vi "testStopServer.vi"(8 "error in (no error)":errorcluster) -> (0 "error out":errorcluster)   [LabVIEW 2018]
doc: "Test the stopServer.vi."
uses:
  src/FactoryTcpServer/FactoryTcpServer.lvclass
  src/TcpServer/TcpServer.lvclass/TcpServer.ctl
  src/TcpServerTel/TcpServerTel.lvclass/TcpServerTel.ctl
  src/TcpServerCmd/TcpServerCmd.lvclass
  home/pcortes/Documents/github/ts_labview_tcp_json/src/TcpServerBase/TcpServerBase.lvclass
  src/TcpServerTel/TcpServerTel.lvclass
  <vilib>/addons/_JKI Toolkits/Caraya/classes/Assert/Assert False.vi
  <vilib>/addons/_JKI Toolkits/Caraya/classes/Assert/Assert True.vi
  <vilib>/addons/_JKI Toolkits/Caraya/classes/Test/Test.lvclass
  <vilib>/addons/_JKI Toolkits/Caraya/classes/Assert/Assert.lvclass
  src/TcpServer/TcpServer.lvclass
  src/TcpServerBase/TcpServerBase.lvclass
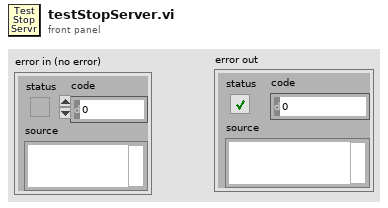
[diagram p1: front panel]
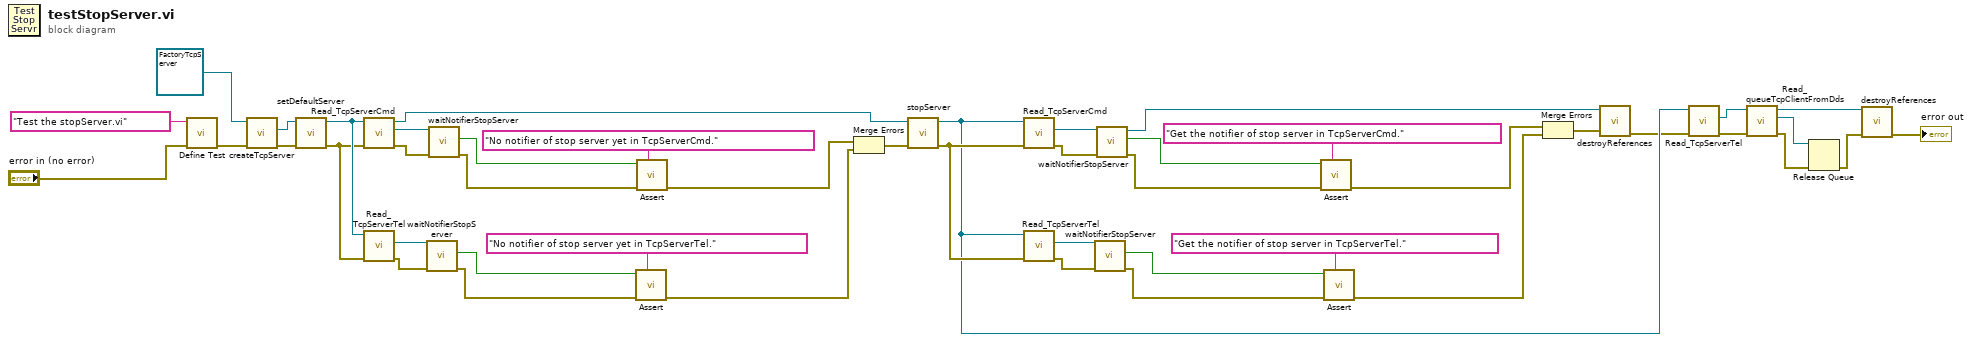
[diagram p0: block diagram]
diagram:
  n1 = call <vilib>:"Define Test.vi"("error in (no error)"="error in (no error)", "Label (VI Title)"="Test the stopServer.vi") -> ("error out"=w15:errorcluster)  [unwired: 9 in]
  n2 = call "createTcpServer.vi"("error in (no error)"=w15, "FactoryTcpServer in"=refnum<class "FactoryTcpServer.lvclass"> refnum) -> ("error out"=w14:errorcluster, "TcpServer out"=w13:refnum<class "TcpServer.lvclass">)  [unwired: 7 in, 1 out]
  n3 = call "setDefaultServer.vi"("error in (no error)"=w14, "TcpServer.lvclass"=w13) -> ("error out"=w42:errorcluster, "tcpServer out"=w43:refnum<class "TcpServer.lvclass">)  [unwired: 8 in]
  n4 = call "Read_TcpServerCmd.vi"("error in (no error)"=w42, "TcpServer in"=w43) -> ("error out"=w39:errorcluster, "TcpServerCmd.lvclass"=w40:refnum<class "TcpServerCmd.lvclass">, "TcpServer out"=w44:refnum<class "TcpServer.lvclass">)  [unwired: 7 in]
  n5 = call "Read_TcpServerTel.vi"("error in (no error)"=w42, "TcpServer in"=w43) -> ("error out"=w37:errorcluster, "TcpServerTel.lvclass"=w38:refnum<class "TcpServerTel.lvclass">)  [unwired: 7 in, 1 out]
  n6 = call "waitNotifierStopServer.vi"("error in (no error)"=w37, "TcpServerBase in"=w38) -> ("error out"=w32:errorcluster, "stopServer"=w33:bool)  [unwired: 7 in, 1 out]
  n7 = call "waitNotifierStopServer.vi"("error in (no error)"=w39, "TcpServerBase in"=w40) -> ("error out"=w31:errorcluster, "stopServer"=w36:bool)  [unwired: 7 in, 1 out]
  n8 = call-poly <vilib>:"Assert.vi"("Label"="No notifier of stop server yet in TcpServerTel.", "error in (no error)"=w32, "False?"=w33) -> ("error out"=w29:errorcluster)  [unwired: 8 in]
  n9 = call-poly <vilib>:"Assert.vi"("Label"="No notifier of stop server yet in TcpServerCmd.", "error in (no error)"=w31, "False?"=w36) -> ("error out"=w30:errorcluster)  [unwired: 8 in]
  n10 = Merge Errors(w30, w29) -> (w41:errorcluster)
  n11 = call "stopServer.vi"("error in (no error)"=w41, "tcpServer in"=w44) -> ("error out"=w22:errorcluster, "tcpServer out"=w7:refnum<class "TcpServer.lvclass">)  [unwired: 8 in]
  n12 = call "Read_TcpServerCmd.vi"("error in (no error)"=w22, "TcpServer in"=w7) -> ("error out"=w20:errorcluster, "TcpServerCmd.lvclass"=w21:refnum<class "TcpServerCmd.lvclass">)  [unwired: 7 in, 1 out]
  n13 = call "Read_TcpServerTel.vi"("error in (no error)"=w22, "TcpServer in"=w7) -> ("error out"=w18:errorcluster, "TcpServerTel.lvclass"=w19:refnum<class "TcpServerTel.lvclass">)  [unwired: 7 in, 1 out]
  n14 = call "waitNotifierStopServer.vi"("error in (no error)"=w18, "TcpServerBase in"=w19) -> ("error out"=w27:errorcluster, "stopServer"=w26:bool)  [unwired: 7 in, 1 out]
  n15 = call "waitNotifierStopServer.vi"("error in (no error)"=w20, "TcpServerBase in"=w21) -> ("error out"=w28:errorcluster, "stopServer"=w23:bool, "TcpServerBase out"=w12:refnum<class "TcpServerCmd.lvclass">)  [unwired: 7 in]
  n16 = call-poly <vilib>:"Assert.vi"("Label"="Get the notifier of stop server in TcpServerCmd.", "error in (no error)"=w28, "True?"=w23) -> ("error out"=w17:errorcluster)  [unwired: 8 in]
  n17 = call-poly <vilib>:"Assert.vi"("Label"="Get the notifier of stop server in TcpServerTel.", "error in (no error)"=w27, "True?"=w26) -> ("error out"=w6:errorcluster)  [unwired: 8 in]
  n18 = Merge Errors(w17, w6) -> (w5:errorcluster)
  n19 = call "destroyReferences.vi"("error in (no error)"=w5, "tcpServerBase in"=w12) -> ("error out"=w4:errorcluster)  [unwired: 8 in, 1 out]
  n20 = call "Read_TcpServerTel.vi"("error in (no error)"=w4, "TcpServer in"=w7) -> ("error out"=w9:errorcluster, "TcpServerTel.lvclass"=w8:refnum<class "TcpServerTel.lvclass">)  [unwired: 7 in, 1 out]
  n21 = call "Read_queueTcpClientFromDds.vi"("error in (no error)"=w9, "TcpServerTel in"=w8) -> ("error out"=w10:errorcluster, "queueTcpClientFromDds"=w11:refnum<queue>, "TcpServerTel out"=w3:refnum<class "TcpServerTel.lvclass">)  [unwired: 7 in]
  n22 = Release Queue(queue=w11, error in (no error)=w10) -> (error out=w2:errorcluster)  [unwired: 1 in, 2 out]
  n23 = call "destroyReferences.vi"("error in (no error)"=w2, "tcpServerBase in"=w3) -> ("error out"=→"error out":errorcluster)  [unwired: 8 in, 1 out]
